vi "Init_DM_DUAL_V2.vi"(7 "BM Flat":bool, 8 "BM Flat File":string[](array[string]), 9 "Control Mode In":string[](array[string]), 10 "DM Mapping File":string, 11 "Base File Path":path) -> (3 "reference out":refnum<k7>)   [LabVIEW 2014]
uses:
  Controls/Standard Action.ctl
  <vilib>/Utility/file.llb/Read From Spreadsheet File (string).vi
  <vilib>/Utility/file.llb/Read From Spreadsheet File (DBL).vi
panel:
  out "IDs":i32[](array[numeric])
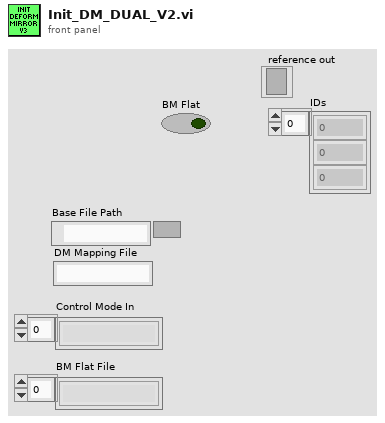
[diagram p1: front panel]
types:
  T1 = typedef "Standard Action.ctl" = enum16{"Read", "Write"}
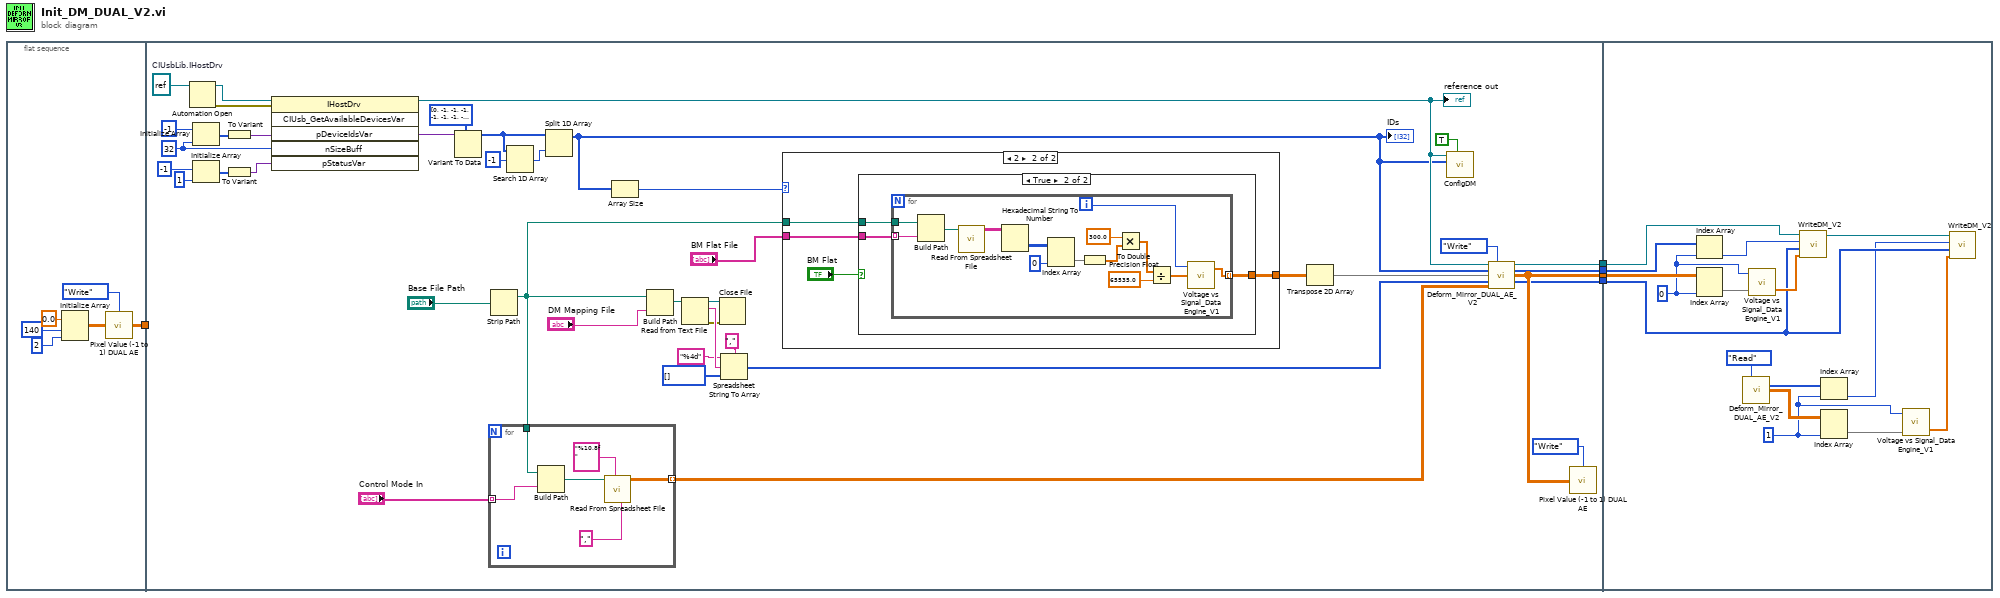
[diagram p0: block diagram]
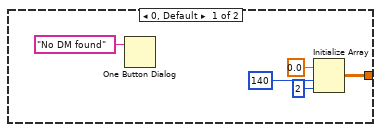
[diagram p2: hidden frame]
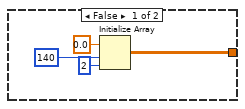
[diagram p3: hidden frame]
diagram:
  n1 = flat-sequence {
    tunnel: [w6] -> w2
    tunnel: [w16] -> w5
    tunnel: [w13] -> w4
    tunnel: [w15] -> w3
    tunnel: w2 -> [_]
    tunnel: [w12] -> w1
    tunnel: w5 -> [w101]
    tunnel: w4 -> [w105]
    tunnel: w3 -> [w103]
    tunnel: w1 -> [w97]
    frame #0 {
      n2 = Initialize Array(0.0 ("element"), 140 ("dimension size"), 2 ("dimension size")) -> (w8:dbl[][])
      n3 = call "Pixel Value (-1 to 1) DUAL AE.vi"("Action"=Standard_Action."Write", "Pixel Value (-1 to 1)"=w8) -> ("Pixel Value (-1 to 1) Out"=w6:dbl[][])  [unwired: 13 in]
    }
    frame #1 {
      w48 = 32 ("dimension size")
      w39 = refnum<k7> refnum  # CIUsbLib.IHostDrv
      n4 = Automation Open(Automation Refnum=w39) -> (Automation Refnum=w44:refnum<k7>, error out=w45:errorcluster)  [unwired: 1 in, 2 out]
      n5 = Initialize Array(-1 ("element"), w48) -> (w41:i32[])
      n6 = Initialize Array(-1 ("element"), 1 ("dimension size")) -> (w40:i32[])
      n7 = To Variant(anything=w41) -> (Variant=w42:variant)
      n8 = To Variant(anything=w40) -> (Variant=w47:variant)
      n9 = invoke class="IHostDrv" method="CIUsb_GetAvailableDevicesVar"(reference=w44, error in=w45, "pDeviceIdsVar"=w42, "nSizeBuff"=w48, "pStatusVar"=w47) -> (reference out=w27:refnum<k7>, "pDeviceIdsVar"=w53:variant)  [unwired: 1 in, 4 out]
      "reference out" <- w27
      n10 = Variant To Data(type=i32[] [0, -1, -1, -1, -1, -1, -1, -1, -1, -1, -1, -1, -1, -1, -1, -1, -1, -1, -1, -1, -1, -1, -1, -1, -1, -1, -1, -1, -1, -1, -1, -1] ("pDeviceIDs"), Variant=w53) -> (data=w51:i32[])  [unwired: 1 in, 1 out]
      n11 = Strip Path(path="Base File Path") -> (stripped path=w31:path)  [unwired: 1 out]
      n12 = for {
        tunnel: w31 -> [w57]
        tunnel: "Control Mode In" -> [w55] mode=indexing
        tunnel: [w54] -> w17 mode=indexing
        n13 = Build Path(base path=w57, name or relative path=w55) -> (appended path=w58:path)
        n14 = call-poly <vilib>:"Read From Spreadsheet File.vi"("delimiter (\\t)"="," ("delimiter (\\t)"), "format (%.3f)"="%10.8f", "file path (dialog if empty)"=w58) -> ("all rows"=w54:dbl[][])  [unwired: 2 in, 6 out]
      }
      n15 = Search 1D Array(1D array=w51, element=-1) -> (index of element=w50:i32)  [unwired: 1 in]
      n16 = Split 1D Array(array=w51, index=w50) -> (first subarray=w20:i32[])  [unwired: 1 out]
      "IDs" <- w20
      n17 = Array Size(array=w20) -> (size(s)=w29:i32)
      n18 = Build Path(base path=w31, name or relative path="DM Mapping File") -> (appended path=w32:path)
      n19 = Read from Text File(file (use dialog)=w32) -> (refnum out=w34:refnum<file>, text=w38:string, error out=w33:errorcluster)  [unwired: 1 in, 3 out]
      n20 = Close File(refnum=w34, error in=w33) -> ()  [unwired: 2 out]
      n21 = Spreadsheet String To Array(delimiter (Tab)=",", format string="%4d", spreadsheet string=w38, array type (2D Dbl)=i32[] []) -> (array=w22:i32[])
      n22 = case shown="2" w29 {
        tunnel: w31 -> [_ w68]
        tunnel: "BM Flat File" -> [_ w67]
        tunnel: [w60 w66] -> w21
        frame 0, Default {
          n23 = One Button Dialog(message="No DM found") -> ()  [unwired: 1 in, 1 out]
          n24 = Initialize Array(0.0 ("element"), 140 ("dimension size"), 2 ("dimension size")) -> (w60:dbl[][])
        }
        frame 2 {
          n25 = case shown="True" "BM Flat" {
            tunnel: w68 -> [_ w75]
            tunnel: w67 -> [_ w73]
            tunnel: [w69 w74] -> w66
            frame False {
              n26 = Initialize Array(0.0 ("element"), 140 ("dimension size"), 2 ("dimension size")) -> (w69:dbl[][])
            }
            frame True {
              n27 = for {
                tunnel: w75 -> [w89]
                tunnel: [w77] -> w74 mode=indexing
                tunnel: w73 -> [w79] mode=indexing
                i -> [w76]
                n28 = Build Path(base path=w89, name or relative path=w79) -> (appended path=w88:path)
                n29 = call-poly <vilib>:"Read From Spreadsheet File.vi"("file path (dialog if empty)"=w88) -> ("all rows"=w87:string[][])  [unwired: 3 in, 7 out]
                n30 = Hexadecimal String To Number(string=w87) -> (number=w86:u32[][])  [unwired: 2 in, 1 out]
                n31 = Index Array(array=w86, index (col)=0 ("disabled index (col)")) -> (element=w84:u32[])  [unwired: 1 in]
                n32 = To Double Precision Float(number=w84) -> (double precision float=w80:dbl[])
                n33 = Multiply(x=300.0 ("y"), y=w80) -> (x*y=w83:dbl[])
                n34 = Divide(x=w83, y=65535.0) -> (x/y=w78:dbl[])
                n35 = call "Voltage vs Signal_Data Engine_V1.vi"("Voltage in (0~Max. Vol.)"=w78, "DM #"=w76) -> ("Control Signal Out (-1~1)"=w77:dbl[])  [unwired: 1 in, 1 out]
              }
            }
          }
        }
      }
      n36 = Transpose 2D Array(2D array=w21) -> (transposed array=w19:dbl[][])
      n37 = call "ConfigDM.vi"("High Voltage"=TRUE, "Dev IDs"=w20, "Automation Refnum in"=w27) -> ()  [unwired: 7 in, 2 out]
      n38 = call "Deform_Mirror_DUAL_AE_V2.vi"("Refnum In"=w27, "Action"=Standard_Action."Write", "IDs In"=w20, "Flat Files In"=w19, "Multi Map Data In"=w22, "Mode Matrix In"=w17) -> ("Refnum Out"=w16:refnum<k7>, "IDs Out"=w15:i32[], "Flat Files Out"=w13:dbl[][], "Multi Map Data Out"=w12:i32[])  [unwired: 5 in, 1 out]
      n39 = call "Pixel Value (-1 to 1) DUAL AE.vi"("Action"=Standard_Action."Write", "Pixel Value (-1 to 1)"=w13) -> ()  [unwired: 13 in, 1 out]
    }
    frame #2 {
      w90 = 1 ("index (col)")
      w102 = 0 ("disabled index (col)")
      n40 = Index Array(array=w103, index=w102) -> (element=w100:i32)
      n41 = Index Array(array=w105, index (col)=w102) -> (element=w104:dbl[])  [unwired: 1 in]
      n42 = call "Deform_Mirror_DUAL_AE_V2.vi"("Action"=Standard_Action."Read") -> ("IDs Out"=w95:i32[], "Flat Files Out"=w94:dbl[][])  [unwired: 10 in, 3 out]
      n43 = call "Voltage vs Signal_Data Engine_V1.vi"("Control Signal In (-1~1)"=w104, "DM #"=w102) -> ("Voltage Out (0~Max. Vol.)"=w99:dbl[])  [unwired: 1 in, 1 out]
      n44 = call "WriteDM_V2.vi"("reference in"=w101, "nDevId"=w100, "MultiDM  Mapping"=w97, "Voltage Array in"=w99) -> ("reference out"=w98:refnum<k7>)  [unwired: 2 in, 1 out]
      n45 = Index Array(array=w95, index=w90) -> (element=w93:i32)
      n46 = Index Array(array=w94, index (col)=w90) -> (element=w92:dbl[])  [unwired: 1 in]
      n47 = call "Voltage vs Signal_Data Engine_V1.vi"("Control Signal In (-1~1)"=w92, "DM #"=w90) -> ("Voltage Out (0~Max. Vol.)"=w91:dbl[])  [unwired: 1 in, 1 out]
      n48 = call "WriteDM_V2.vi"("reference in"=w98, "nDevId"=w93, "MultiDM  Mapping"=w97, "Voltage Array in"=w91) -> ()  [unwired: 2 in, 2 out]
    }
  }
